vi "Undistort Image.vi"   [LabVIEW 2020, in "ar.lvlib" / "Image Undistorter.lvclass"]
doc: "Undistort the Source Image. The Destination image will be sized to fit."
uses:
  Image Undistorter.lvclass
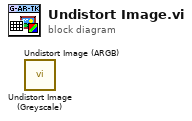
[diagram p0: block diagram]
diagram:
  n1 = call "Undistort Image (Greyscale).vi"() -> ()  [unwired: 9 in, 3 out]
  n2 = call "Undistort Image (ARGB).vi"() -> ()  [unwired: 9 in, 3 out]
